vi "TCP Reception Initialization.vi"(11 "Camera Streams":i32) -> (3 "Cluster":T2)   [LabVIEW 2015]
uses:
  <vilib>/vision/Image Controls.llb/IMAQ Image.ctl
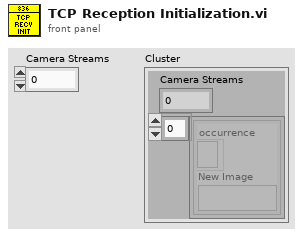
[diagram p1: front panel]
types:
  T1 = typedef "IMAQ Image.ctl" = refnum<image>
  T2 = cluster{"Camera Streams":i32, cluster{"occurrence":refnum<k4>, "New Image":T1}[]}
  T3 = typedef "Image Type" = u32
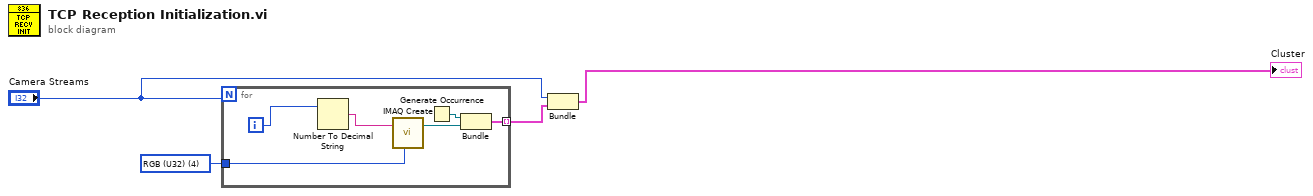
[diagram p0: block diagram]
diagram:
  w1 = T3 4 items=["Grayscale (U8)", "Grayscale (I16)", "Grayscale (SGL)", "Complex (CSG)", "RGB (U32)", "HSL (U32)", "RGB (U64)", "Grayscale (U16)"] ("Image Type")
  n1 = for {
    N: "Camera Streams" -> [_]
    tunnel: w1 -> [w10]
    tunnel: [w7] -> w2 mode=indexing
    i -> [w6]
    n2 = Number To Decimal String(number=w6) -> (decimal integer string=w5:string)  [unwired: 1 in]
    n3 = call "IMAQ Create"("Image Name"=w5, "Image Type"=w10) -> ("New Image"=w8:T1)  [unwired: 3 in, 1 out]
    n4 = Generate Occurrence() -> (w9:refnum<k4>)
    n5 = Bundle("occurrence"=w9, "New Image"=w8) -> (w7:cluster{"occurrence":refnum<k4>, "New Image":T1})  [unwired: 1 in]
  }
  n6 = Bundle("Camera Streams"="Camera Streams", w2) -> (→"Cluster":T2)  [unwired: 1 in]
